vi "BehaviorEphys.vi"() -> ()   [LabVIEW 2010]
uses:
  TimeStamper/TimeStamper.lvclass
  Electrophysiology/Electrophysiology.lvclass
panel:
  in  "Recording Channels":refnum<k21>="All4498"
  in  "Stream To":string="localhost"
  out "MSamples":dbl
  in  "Audio":cluster{"Left channel":i32, "Right channel":i32}
  in  "Stream channels":i32[](array[numeric])
  in  "Volume":dbl(slide) scale=0.0..5000.0
  in  "Enable Sound":bool
  out "Message":cluster{"Channel":dbl, "Message":string}
  out "Messages":T1(array[cluster])
  in  "Subject":string(combo)="Woody"
  in  "stop":bool
  in  "Root Path":path=path "M:/"
  in  "Counter Card":tag="Dev1"
  in  "Sample Lines":tag[](array[tag])=["/PXI1Slot10/ai/StartTrigger", "/Dev3/ai/StartTrigger", "/Dev1/PFI18"]
  out "Timestamps":u64[][](array[numeric])
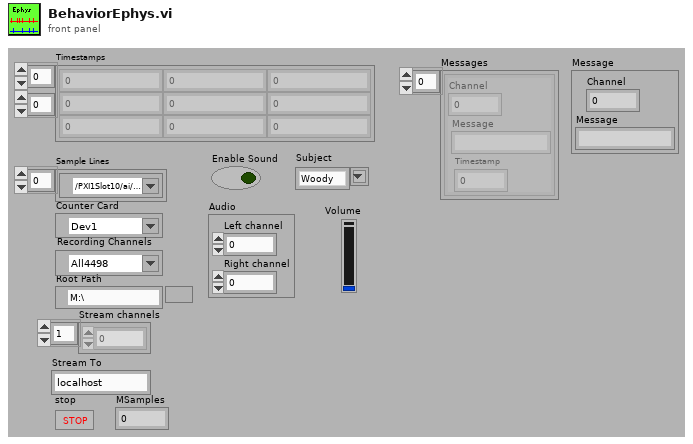
[diagram p1: front panel]
types:
  T1 = cluster{"Channel":dbl, "Message":string, "Timestamp":u64}[]
  T2 = cluster{"Channel":dbl, "Message":string, timestamp}[]
  T3 = cluster{"Channel":i32, "Counter":u32, "Time Stamp":timestamp}[]
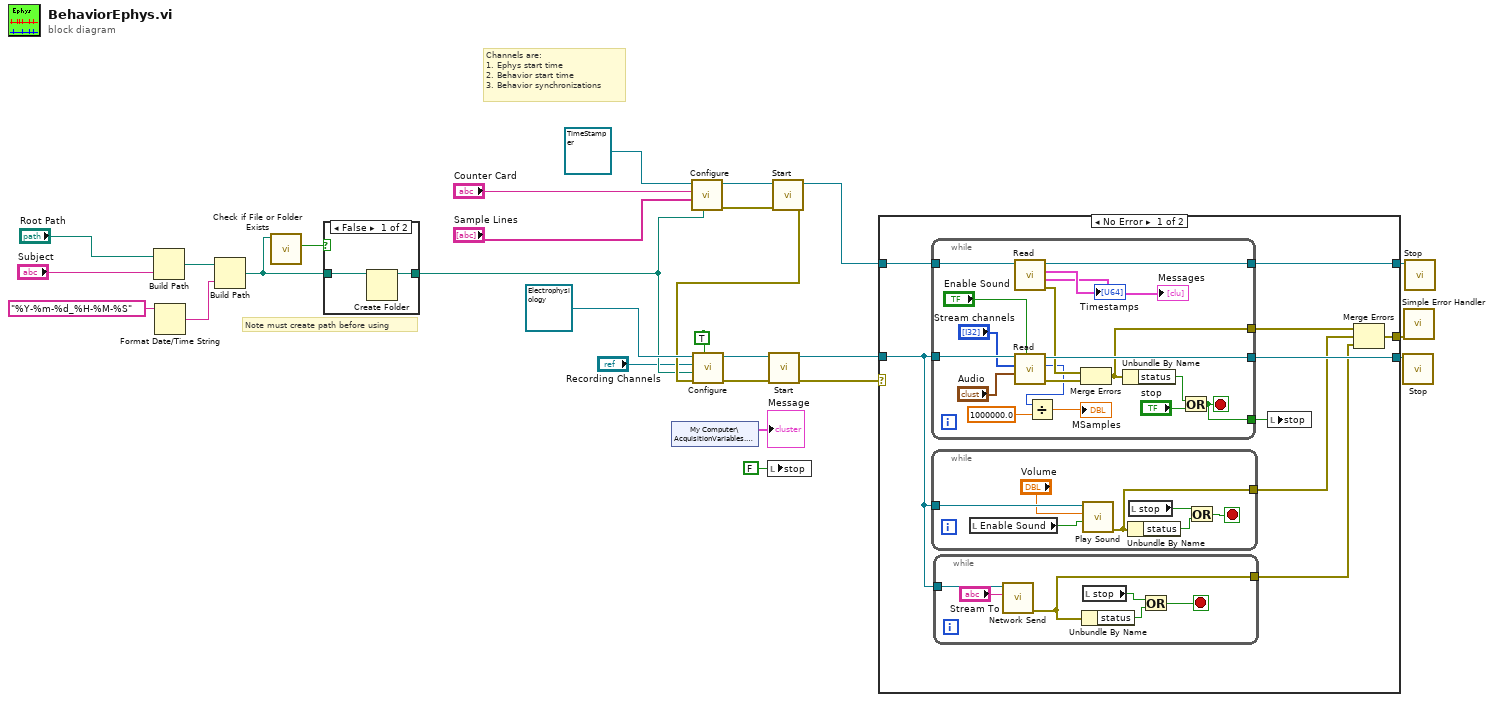
[diagram p0: block diagram]
diagram:
  # "Note must create path before using"
  # "Channels are:\n1. Ephys start time\n2. Behavior start time\n3. Behavior synchronizations"
  n1 = Build Path(base path="Root Path", name or relative path="Subject") -> (appended path=w13:path)
  n2 = Format Date/Time String(time format string (%c)="%Y-%m-%d_%H-%M-%S") -> (date/time string=w8:string)  [unwired: 2 out]
  n3 = Build Path(base path=w13, name or relative path=w8) -> (appended path=w7:path)
  n4 = call <vilib>:"Check if File or Folder Exists.vi"("path"=w7) -> ("file or folder exists?"=w12:bool)  [unwired: 1 in, 9 out]
  n5 = case shown="False" w12 {
    tunnel: w7 -> [w29 w30]
    tunnel: [w28 w30] -> w6
    frame False {
      n6 = Create Folder(path (use dialog)=w29) -> (created path=w28:path)  [unwired: 2 in, 2 out]
    }
    frame True {
    }
  }
  n7 = shared-variable "My Computer\\AcquisitionVariables.lvlib\\Message"() -> (→"Message":cluster{"Channel":dbl, "Message":string})  [unwired: 1 in, 1 out]
  n8 = call-dynamic "Configure.vi"(6:w6, "Sample Lines"="Sample Lines", "DAQmx Device Name"="Counter Card", "TimeStamper in"=refnum<class "TimeStamper.lvclass"> refnum ("TimeStamper.lvclass")) -> ("error out"=w23:errorcluster, "TimeStamper out"=w24:refnum<class "TimeStamper.lvclass">)  [unwired: 6 in]
  n9 = local write "stop"(FALSE ("stop")) -> ()
  n10 = call-dynamic "Start.vi"("error in (no error)"=w23, "TimeStamper in"=w24) -> ("error out"=w17:errorcluster, "TimeStamper out"=w22:refnum<class "TimeStamper.lvclass">)  [unwired: 8 in]
  n11 = call-dynamic "Configure.vi"(7:TRUE ("Enable Sound"), "error in (no error)"=w17, 9:w6, "Recording Channels"="Recording Channels", "Electrophysiology in"=refnum<class "Electrophysiology.lvclass"> refnum ("Electrophysiology.lvclass")) -> ("error out"=w18:errorcluster, "Electrophysiology out"=w19:refnum<class "Electrophysiology.lvclass">)  [unwired: 5 in]
  n12 = call-dynamic "Start.vi"("error in (no error)"=w18, "Electrophysiology in"=w19) -> ("error out"=w14:errorcluster, "Electrophysiology out"=w16:refnum<class "Electrophysiology.lvclass">)  [unwired: 8 in]
  n13 = case shown="No Error" w14 {
    selector: w14 -> [_ w71]
    tunnel: w22 -> [w39 w73]
    tunnel: [w38 w73] -> w21
    tunnel: w16 -> [w36 w72]
    tunnel: [w37 w72] -> w15
    tunnel: [w31 w71] -> w1
    frame No Error {
      n14 = while {
        tunnel: w39 -> [w70]
        tunnel: [w69] -> w38
        tunnel: w36 -> [w67]
        tunnel: [w66] -> w37
        tunnel: [w54] -> w34
        tunnel: [w53] -> w35
        stop <- w53 stop-if-true
        n15 = call-dynamic "Read.vi"("TimeStamper in"=w70) -> ("error out"=w63:errorcluster, "Messages"=→"Messages":T2, "Timestamps"=→"Timestamps":T3, "TimeStamper out"=w69:refnum<class "TimeStamper.lvclass">)  [unwired: 7 in]
        n16 = call-dynamic "Read.vi"("Enable Sound"="Enable Sound", "Audio Channels"="Audio", 10:"Stream channels", "Electrophysiology in"=w67) -> ("error out"=w64:errorcluster, "Samples"=w57:u32, "Electrophysiology out"=w66:refnum<class "Electrophysiology.lvclass">)  [unwired: 5 in]
        n17 = Divide(x=w57, y=1000000.0) -> (x/y=→"MSamples":dbl)
        n18 = Merge Errors(w63, w64) -> (w54:errorcluster)
        n19 = Unbundle By Name(w54) -> ("status"=w62:bool)
        n20 = Or(x=w62, y="stop") -> (x .or. y?=w53:bool)
      }
      n21 = while {
        tunnel: w36 -> [w52]
        tunnel: [w46] -> w33
        stop <- w49 stop-if-true
        n22 = local read "Enable Sound"() -> (w47:bool)
        n23 = call-dynamic "Play Sound.vi"("Enable Sound"=w47, "Volume"="Volume", "Electrophysiology in"=w52) -> ("error out"=w46:errorcluster)  [unwired: 7 in, 1 out]
        n24 = Unbundle By Name(w46) -> ("status"=w50:bool)
        n25 = local read "stop"() -> (w51:bool)
        n26 = Or(x=w51, y=w50) -> (x .or. y?=w49:bool)
      }
      n27 = while {
        tunnel: w36 -> [w45]
        tunnel: [w40] -> w32
        stop <- w42 stop-if-true
        n28 = call-dynamic "Network Send.vi"("Target IP Address"="Stream To", "Electrophysiology in"=w45) -> ("error out"=w40:errorcluster)  [unwired: 8 in, 1 out]
        n29 = Unbundle By Name(w40) -> ("status"=w43:bool)
        n30 = local read "stop"() -> (w44:bool)
        n31 = Or(x=w44, y=w43) -> (x .or. y?=w42:bool)
      }
      n32 = local write "stop"(w35) -> ()
      n33 = Merge Errors(w34, w33, w32) -> (w31:errorcluster)
    }
    frame Error {
    }
  }
  n34 = call-dynamic "Stop.vi"("Electrophysiology in"=w15) -> ()  [unwired: 9 in, 2 out]
  n35 = call <vilib>:"Simple Error Handler.vi"("error in (no error)"=w1) -> ()  [unwired: 4 in, 5 out]
  n36 = call-dynamic "Stop.vi"("TimeStamper in"=w21) -> ()  [unwired: 9 in, 2 out]
